vi "Selected Doc Object[].vi"(0 "Doc Class Object[]":refnum<class "Document.lvclass">[](array[class]), 5 "Doc Name[]":string[](array[string]), 11 "error in":errorcluster) -> (4 "Selected Doc[]":refnum<class "Document.lvclass">[](array[class]), 15 "error Out":errorcluster)   [LabVIEW 2016, in "LV MDI.lvclass"]
uses:
  LV MDI.lvclass
  Document/Document.lvclass
  Document/Document.lvclass/Document.ctl
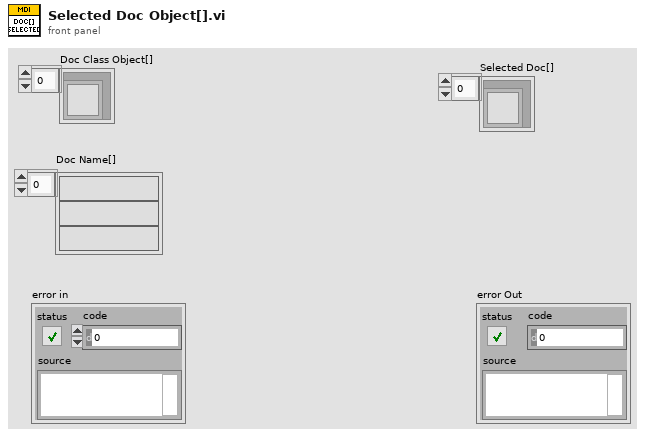
[diagram p1: front panel]
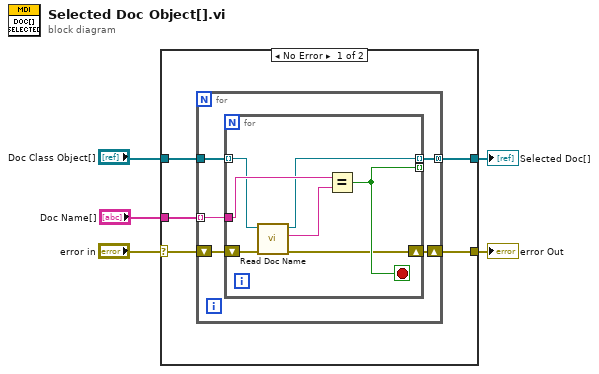
[diagram p0: block diagram]
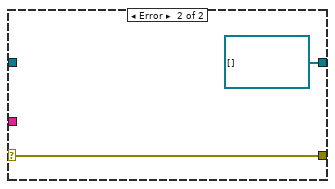
[diagram p2: hidden frame]
diagram:
  n1 = case shown="No Error" "error in" {
    selector: "error in" -> [w7 w23]
    tunnel: [w10 refnum<class "Document.lvclass">[] []] -> w1
    tunnel: "Doc Class Object[]" -> [w9 _]
    tunnel: "Doc Name[]" -> [w8 _]
    tunnel: [w6 w23] -> w2
    frame No Error {
      n2 = for {
        tunnel: w9 -> [w14]
        tunnel: w8 -> [w15] mode=indexing
        tunnel: [w13] -> w10 mode=concatenating
        shift-right: [w11] -> w6
        shift-left: w7 -> [w12]
        n3 = for {
          tunnel: w15 -> [w19]
          tunnel: w14 -> [w17] mode=indexing
          tunnel: [w16] -> w13 mode=indexing if=w22
          tunnel: [w22] -> _ mode=indexing
          shift-right: [w20] -> w11
          shift-left: w12 -> [w21]
          stop <- w22 stop-if-true
          n4 = call "Read Doc Name.vi"("error in (no error)"=w21, "Document in"=w17) -> ("error out"=w20:errorcluster, "Doc Name"=w18:string, "Document out"=w16:refnum<class "Document.lvclass">)  [unwired: 7 in]
          n5 = Equal?(x=w19, y=w18) -> (x = y?=w22:bool)
        }
      }
    }
    frame Error {
    }
  }
  "error Out" <- w2
  "Selected Doc[]" <- w1
